vi "FocusLock Control v3.vi"() -> ()   [LabVIEW 2014]
uses:
  Controls/Camera Control.ctl
  Controls/Focus Lock.ctl
  Controls/Standard Action for Camera Control.ctl
  Controls/Standard Action for Focus Lock.ctl
  Controls/Counter Action.ctl
  Controls/Standard Action for Position.ctl
  Controls/StageStates.ctl
  <vilib>/addons/control/pid/pid.llb/PID (DBL Array).vi
  <vilib>/Utility/xml.llb/Write to XML File(string).vi
  <vilib>/Utility/xml.llb/Read From XML File(string).vi
  C:/Program Files (x86)/National Instruments/LabVIEW 2014/instr.lib/IDS/ueye.NET/uEyeDotNet.dll
  Program Files (x86)/National Instruments/LabVIEW 2014/instr.lib/IDS/ueye.NET/uEyeDotNet.dll
  <vilib>/addons/control/pid/NI_PID_pid.lvlib
panel:
  in  "Load":bool
  in  "Save":bool
  out "metric":dbl[](array[numeric])
  in  "Lock Control":T1
  out "Lock Position":cluster{"X":dbl, "Y":dbl, "dx - dy":dbl}
  out "Current Position":cluster{"X":dbl, "Y":dbl, "dx - dy":dbl}
  out "Size difference History":dbl(graph)
  out "Position History":cluster{dbl, dbl}(graph)
  in  "Lock Tolorence":cluster{"XY":dbl, "Z":dbl}={"XY"=0.4, "Z"=0.4}
  out "ROI":u8[][](graph)=[[1, 1, 1, 1, 1, 1, 1, 1, 1, 2, 1, 1, 1, 1, 1, 2, 1, 1, 1, 1, 1, 2, 1, 1, 1, 1, 1, 1, 1, 1, 1, 1, 1, 1, 1, 1, 1, 1, 1, 1, 1, 1, 1, 1, 1, 1, 1, 1, 1, 1], [0, 1, 1, 1, 1, 1, 1, 1, 0, 1, 0, 1, 0, 1, 0, 1, 0, 1, 0, 1, 0, 1, 0, 1, 0, 1, 0, 1, 0, 1, 1, 1, 0, 1, 0, 1, 0, 1, 0, 1, 0, 1, 0, 1, 0, 1, 0, 1, 0, 1], [1, 1, 1, 1, 1, 1, 1, 1, 1, 1, 1, 1, 1, 1, 1, 1, 1, 2, 1, 1, 1, 1, 1, 1, 1, 1, 1, 1, 1, 1, 1, 1, 1, 1, 1, 1, 1, 1, 1, 1, 1, 1, 1, 1, 1, 1, 1, 1, 1, 1], [0, 1, 1, 1, 1, 1, 0, 1, 0, 1, 0, 1, 0, 1, 0, 1, 0, 1, 0, 1, 0, 1, 0, 1, 0, 1, 0, 1, 0, 1, 0, 1, 0, 1, 0, 1, 0, 1, 0, 1, 0, 1, 0, 1, 0, 1, 0, 1, 0, 1], [1, 1, 1, 1, 1, 1, 1, 1, 1, 1, 1, 1, 1, 1, 1, 1, 1, 1, 1, 1, 1, 1, 1, 1, 1, 1, 1, 1, 1, 1, 1, 1, 1, 1, 1, 1, 1, 1, 1, 1, 1, 1, 1, 1, 1, 1, 1, 1, 1, 2], [0, 1, 0, 1, 0, 1, 0, 1, 0, 1, 0, 1, 0, 1, 1, 1, 0, 1, 0, 1, 0, 1, 0, 1, 0, 1, 1, 1, 0, 1, 1, 1, 0, 1, 0, 1, 0, 1, 1, 1, 0, 1, 0, 1, 0, 1, 0, 1, 0, 1], [1, 1, 1, 1, 1, 2, 1, 1, 1, 1, 1, 1, 1, 2, 1, 2, 1, 1, 1, 2, 1, 2, 1, 1, 1, 1, 1, 1, 1, 1, 1, 2, 1, 1, 1, 2, 1, 2, 1, 1, 1, 1, 1, 1, 1, 2, 1, 1, 1, 2], [0, 1, 0, 1, 0, 1, 0, 1, 1, 1, 1, 1, 0, 1, 0, 1, 0, 1, 0, 1, 0, 1, 0, 1, 0, 1, 0, 1, 0, 1, 0, 1, 0, 1, 0, 1, 0, 1, 1, 1, 1, 1, 0, 1, 0, 1, 0, 1, 0, 1], [1, 1, 1, 2, 1, 2, 1, 1, 1, 2, 1, 1, 1, 1, 1, 1, 1, 1, 1, 1, 1, 2, 1, 1, 1, 2, 1, 1, 1, 1, 1, 1, 1, 1, 1, 1, 1, 1, 1, 1, 1, 1, 1, 1, 1, 1, 1, 2, 1, 1], [0, 1, 1, 1, 0, 1, 0, 1, 0, 1, 0, 1, 0, 1, 1, 1, 0, 1, 0, 1, 0, 1, 0, 1, 1, 1, 0, 1, 0, 1, 1, 1, 0, 1, 0, 1, 1, 1, 0, 1, 0, 1, 0, 1, 0, 1, 0, 1, 0, 1], [1, 1, 1, 1, 1, 1, 1, 1, 1, 1, 1, 2, 1, 2, 1, 1, 1, 1, 1, 1, 1, 1, 1, 1, 1, 1, 1, 1, 1, 1, 1, 1, 1, 1, 1, 1, 1, 1, 1, 1, 1, 2, 1, 1, 1, 1, 1, 2, 1, 1], [1, 1, 0, 1, 1, 1, 1, 1, 1, 1, 1, 1, 1, 1, 0, 1, 0, 1, 1, 1, 1, 1, 1, 1, 1, 1, 1, 1, 1, 1, 0, 1, 0, 1, 1, 1, 1, 1, 0, 1, 1, 1, 1, 1, 0, 1, 0, 1, 0, 1], [1, 1, 1, 1, 1, 1, 1, 1, 1, 2, 1, 1, 1, 1, 1, 1, 1, 1, 1, 1, 1, 1, 1, 2, 1, 1, 1, 2, 1, 2, 1, 1, 1, 2, 1, 1, 1, 1, 1, 1, 1, 2, 1, 1, 1, 1, 1, 2, 1, 1], [0, 1, 0, 1, 1, 1, 0, 1, 1, 1, 1, 1, 1, 1, 1, 1, 1, 1, 0, 1, 0, 1, 0, 1, 0, 1, 1, 1, 1, 1, 0, 1, 0, 1, 1, 1, 0, 1, 0, 1, 1, 1, 1, 1, 0, 1, 1, 1, 0, 1], [1, 1, 1, 1, 1, 1, 1, 2, 1, 1, 1, 2, 1, 1, 1, 1, 1, 1, 1, 1, 1, 1, 1, 2, 1, 2, 1, 1, 1, 1, 1, 1, 1, 1, 1, 1, 1, 1, 1, 1, 1, 1, 1, 1, 1, 1, 1, 2, 1, 1], [0, 1, 0, 1, 1, 1, 1, 1, 0, 1, 0, 1, 0, 1, 0, 1, 1, 1, 0, 1, 0, 1, 0, 1, 0, 1, 0, 1, 0, 1, 0, 1, 0, 1, 0, 1, 0, 1, 0, 1, 1, 1, 0, 1, 1, 1, 0, 1, 1, 1], [1, 1, 1, 1, 1, 1, 1, 1, 1, 2, 1, 1, 1, 1, 1, 1, 1, 1, 1, 1, 1, 1, 1, 1, 1, 1, 1, 1, 1, 2, 1, 2, 1, 1, 1, 1, 1, 1, 1, 1, 1, 1, 1, 1, 1, 1, 1, 1, 1, 1], [0, 1, 0, 1, 1, 1, 0, 1, 0, 1, 0, 1, 0, 1, 0, 1, 1, 1, 0, 1, 0, 1, 0, 1, 0, 1, 0, 1, 0, 1, 0, 1, 0, 1, 0, 1, 0, 1, 0, 1, 0, 1, 0, 1, 0, 1, 0, 1, 0, 1], [1, 1, 1, 1, 1, 1, 1, 2, 1, 1, 1, 1, 1, 1, 1, 1, 1, 1, 1, 1, 1, 1, 1, 1, 1, 2, 1, 1, 1, 1, 1, 1, 1, 1, 1, 1, 1, 1, 1, 2, 1, 2, 1, 1, 1, 2, 1, 2, 1, 2], [0, 1, 1, 1, 0, 1, 0, 1, 0, 1, 0, 1, 0, 1, 0, 1, 1, 1, 0, 1, 0, 1, 0, 1, 0, 1, 0, 1, 0, 1, 1, 1, 0, 1, 0, 1, 0, 1, 0, 1, 0, 1, 0, 1, 0, 1, 0, 1, 0, 1], [1, 2, 1, 1, 1, 1, 1, 1, 1, 1, 1, 1, 1, 1, 1, 1, 1, 2, 1, 1, 1, 1, 1, 1, 1, 2, 1, 1, 1, 2, 1, 2, 1, 2, 1, 1, 1, 1, 1, 2, 1, 1, 1, 2, 1, 2, 1, 1, 1, 1], [0, 1, 0, 1, 1, 1, 0, 1, 0, 1, 0, 1, 1, 1, 0, 1, 0, 1, 0, 1, 0, 1, 0, 1, 0, 1, 0, 1, 0, 1, 0, 1, 0, 1, 0, 1, 0, 1, 0, 1, 0, 1, 0, 1, 0, 1, 0, 1, 0, 1], [1, 1, 1, 1, 1, 1, 1, 1, 1, 2, 1, 1, 1, 1, 1, 1, 1, 1, 1, 1, 1, 1, 1, 1, 1, 1, 1, 1, 1, 1, 1, 1, 1, 1, 1, 1, 1, 2, 1, 1, 1, 2, 1, 1, 1, 1, 1, 1, 1, 1], [0, 1, 0, 1, 0, 1, 1, 1, 0, 1, 0, 1, 0, 1, 0, 1, 0, 1, 0, 1, 0, 1, 0, 1, 0, 1, 0, 1, 0, 1, 0, 1, 0, 1, 0, 1, 0, 1, 1, 1, 0, 1, 0, 1, 0, 1, 1, 1, 1, 1], [1, 1, 1, 1, 1, 1, 1, 1, 1, 1, 1, 1, 1, 1, 1, 1, 1, 2, 1, 2, 1, 1, 1, 1, 1, 1, 1, 2, 1, 1, 1, 1, 1, 2, 1, 2, 1, 1, 1, 1, 1, 1, 1, 1, 1, 1, 1, 1, 1, 2], [1, 1, 0, 1, 0, 1, 0, 1, 1, 1, 0, 1, 0, 1, 0, 1, 1, 1, 0, 1, 0, 1, 0, 1, 1, 1, 1, 1, 1, 1, 0, 1, 1, 1, 1, 1, 1, 1, 1, 1, 0, 1, 1, 1, 0, 1, 0, 1, 0, 1], [1, 1, 1, 1, 1, 1, 1, 1, 1, 1, 1, 1, 1, 1, 1, 2, 1, 1, 1, 1, 1, 1, 1, 1, 1, 1, 1, 1, 1, 1, 1, 1, 1, 1, 1, 1, 1, 1, 1, 1, 1, 1, 1, 1, 1, 1, 1, 1, 1, 1], [1, 1, 1, 1, 1, 1, 0, 1, 1, 1, 1, 1, 1, 1, 1, 1, 1, 1, 1, 1, 1, 1, 0, 1, 1, 1, 1, 1, 1, 1, 1, 1, 1, 1, 1, 1, 0, 1, 1, 1, 1, 1, 1, 1, 1, 1, 1, 1, 1, 1], [1, 1, 1, 1, 1, 1, 1, 1, 1, 1, 1, 1, 1, 2, 1, 2, 1, 1, 1, 1, 1, 1, 1, 1, 1, 1, 1, 1, 1, 1, 1, 1, 1, 2, 1, 1, 1, 1, 1, 1, 1, 2, 1, 1, 1, 1, 1, 1, 1, 1], [1, 1, 0, 1, 1, 1, 1, 1, 0, 1, 0, 1, 0, 1, 1, 1, 1, 1, 1, 1, 0, 1, 0, 1, 0, 1, 0, 1, 1, 1, 0, 1, 0, 1, 0, 1, 0, 1, 0, 1, 0, 1, 0, 1, 0, 1, 1, 1, 0, 1], [1, 1, 1, 1, 1, 1, 1, 1, 1, 1, 1, 1, 1, 2, 1, 1, 1, 1, 1, 1, 1, 1, 1, 2, 1, 1, 1, 2, 1, 1, 1, 1, 1, 1, 1, 1, 1, 1, 1, 1, 1, 1, 1, 2, 1, 1, 1, 1, 1, 2], [0, 1, 0, 1, 0, 1, 1, 1, 0, 1, 0, 1, 0, 1, 1, 1, 0, 1, 0, 1, 0, 1, 0, 1, 0, 1, 1, 1, 0, 1, 1, 1, 0, 1, 0, 1, 0, 1, 1, 1, 1, 1, 0, 1, 1, 1, 1, 1, 1, 1], [1, 2, 1, 1, 1, 2, 1, 2, 1, 2, 1, 1, 1, 2, 1, 1, 1, 1, 1, 1, 1, 1, 1, 1, 1, 1, 1, 1, 1, 2, 1, 1, 1, 1, 1, 1, 1, 2, 1, 1, 1, 1, 1, 1, 1, 1, 1, 1, 1, 1], [0, 1, 0, 1, 0, 1, 0, 1, 1, 1, 1, 1, 1, 1, 1, 1, 1, 1, 0, 1, 0, 1, 0, 1, 0, 1, 0, 1, 0, 1, 0, 1, 0, 1, 0, 1, 0, 1, 0, 1, 0, 1, 1, 1, 0, 1, 0, 1, 0, 1], [1, 1, 1, 1, 1, 1, 1, 1, 1, 1, 1, 1, 1, 1, 1, 1, 1, 1, 1, 2, 1, 2, 1, 1, 1, 1, 1, 1, 1, 1, 1, 1, 1, 1, 1, 1, 1, 1, 1, 1, 1, 1, 1, 1, 1, 1, 1, 1, 1, 1], [0, 1, 1, 1, 1, 1, 0, 1, 0, 1, 0, 1, 1, 1, 0, 1, 0, 1, 0, 1, 1, 1, 0, 1, 0, 1, 0, 1, 0, 1, 0, 1, 0, 1, 0, 1, 0, 1, 1, 1, 0, 1, 0, 1, 0, 1, 0, 1, 1, 1], [1, 1, 1, 1, 1, 1, 1, 1, 1, 1, 1, 1, 1, 1, 1, 1, 1, 1, 1, 1, 1, 1, 1, 1, 1, 2, 1, 1, 1, 2, 1, 1, 1, 1, 1, 2, 1, 2, 1, 2, 1, 1, 1, 1, 1, 1, 1, 1, 1, 1], [0, 1, 1, 1, 1, 1, 0, 1, 0, 1, 0, 1, 1, 1, 0, 1, 0, 1, 0, 1, 0, 1, 0, 1, 0, 1, 0, 1, 1, 1, 1, 1, 0, 1, 0, 1, 0, 1, 1, 1, 0, 1, 1, 1, 0, 1, 0, 1, 0, 1], [1, 1, 1, 1, 1, 1, 1, 1, 1, 1, 1, 1, 1, 1, 1, 1, 1, 1, 1, 1, 1, 1, 1, 2, 1, 1, 1, 2, 1, 1, 1, 2, 1, 1, 1, 2, 1, 1, 1, 2, 1, 1, 1, 1, 1, 1, 1, 1, 1, 1], [0, 1, 0, 1, 0, 1, 0, 1, 0, 1, 1, 1, 0, 1, 0, 1, 0, 1, 1, 1, 0, 1, 0, 1, 0, 1, 1, 1, 1, 1, 1, 1, 0, 1, 0, 1, 1, 1, 0, 1, 0, 1, 0, 1, 1, 1, 1, 1, 1, 1], [1, 1, 1, 1, 1, 1, 1, 1, 1, 1, 2, 1, 1, 1, 1, 1, 1, 1, 1, 1, 2, 1, 1, 1, 1, 1, 1, 1, 1, 1, 1, 1, 1, 1, 1, 1, 1, 1, 1, 1, 1, 1, 1, 1, 1, 1, 1, 1, 1, 1], [1, 1, 0, 1, 0, 1, 0, 1, 0, 1, 0, 1, 1, 1, 0, 1, 0, 1, 0, 1, 0, 1, 1, 1, 0, 1, 0, 1, 0, 1, 0, 1, 0, 1, 0, 1, 0, 1, 0, 1, 0, 1, 0, 1, 0, 1, 0, 1, 0, 1], [1, 1, 1, 1, 1, 1, 1, 1, 1, 1, 1, 1, 1, 1, 1, 1, 1, 1, 1, 1, 1, 1, 1, 1, 1, 1, 1, 1, 1, 1, 1, 1, 1, 1, 1, 1, 1, 1, 1, 1, 1, 1, 1, 1, 1, 1, 1, 2, 1, 1], [0, 1, 1, 1, 0, 1, 0, 1, 0, 1, 0, 1, 0, 1, 0, 1, 0, 1, 0, 1, 0, 1, 0, 1, 0, 1, 0, 1, 0, 1, 0, 1, 0, 1, 0, 1, 0, 1, 0, 1, 0, 1, 0, 1, 0, 1, 0, 1, 0, 1], [1, 1, 1, 1, 1, 1, 1, 1, 1, 1, 1, 1, 1, 1, 1, 1, 1, 1, 1, 1, 1, 1, 1, 1, 1, 1, 1, 1, 1, 1, 1, 1, 1, 1, 1, 1, 1, 1, 1, 1, 1, 1, 1, 1, 1, 1, 1, 1, 1, 2], [0, 1, 0, 1, 0, 1, 0, 1, 0, 1, 0, 1, 0, 1, 0, 1, 0, 1, 1, 1, 0, 1, 0, 1, 0, 1, 0, 1, 0, 1, 0, 1, 0, 1, 0, 1, 0, 1, 0, 1, 0, 1, 0, 1, 0, 1, 0, 1, 0, 1], [1, 1, 1, 1, 1, 1, 1, 1, 1, 1, 1, 1, 1, 1, 1, 1, 1, 1, 1, 1, 1, 1, 1, 1, 1, 1, 1, 2, 1, 2, 1, 2, 1, 1, 1, 1, 1, 1, 1, 2, 1, 1, 1, 1, 1, 1, 1, 1, 1, 1], [0, 1, 0, 1, 0, 1, 0, 1, 0, 1, 0, 1, 0, 1, 0, 1, 0, 1, 0, 1, 0, 1, 0, 1, 0, 1, 0, 1, 0, 1, 0, 1, 0, 1, 0, 1, 0, 1, 0, 1, 0, 1, 0, 1, 0, 1, 0, 1, 0, 1], [1, 1, 1, 1, 1, 1, 1, 1, 1, 1, 1, 1, 1, 1, 1, 2, 1, 1, 1, 1, 1, 1, 1, 1, 1, 1, 1, 1, 1, 2, 1, 1, 1, 2, 1, 1, 1, 1, 1, 2, 1, 1, 1, 1, 1, 1, 1, 2, 1, 1], [0, 1, 0, 1, 0, 1, 0, 1, 0, 1, 1, 1, 0, 1, 0, 1, 0, 1, 0, 1, 0, 1, 0, 1, 0, 1, 0, 1, 1, 1, 0, 1, 0, 1, 0, 1, 0, 1, 1, 1, 0, 1, 1, 1, 0, 1, 0, 1, 1, 1]]
  in  "Camera Control":T2={"Pixel Clock (MHz)"=0, "Exposure Time (ms)"=0.0, "Frame Rate (fps)"=10.000850072256142, "ROI Half Width"=100, "Switch"=TRUE} {"Frame Rate (fps)" scale=6.1..17.45; "Exposure Time (ms)" scale=0.06..1.0; "Pixel Clock (MHz)" scale=5.0..43.0}
  out "Camera Image":u8[][](graph)
  in  "Laser Control":refnum<k7>(container)
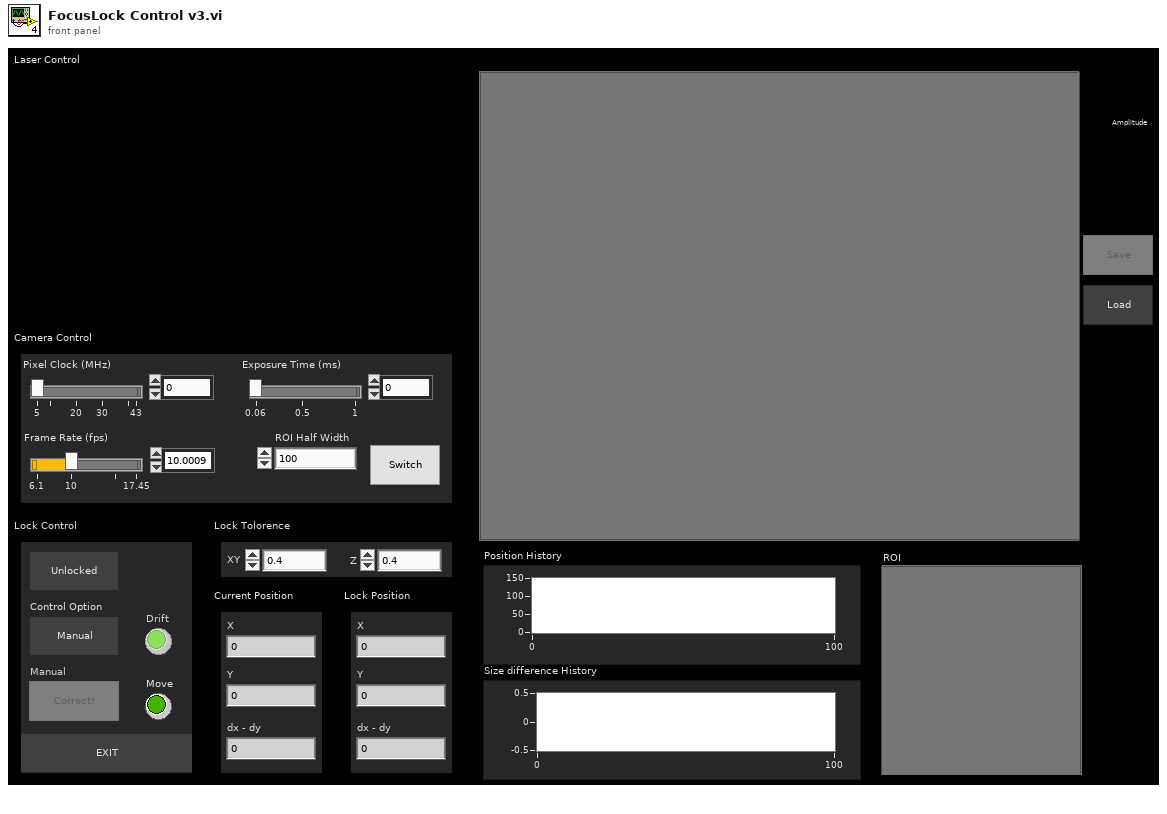
[diagram p1: front panel]
types:
  T1 = typedef "Focus Lock.ctl" = cluster{"EXIT":bool, "Lock Current":bool, "Manual":bool, "Drift":bool, "Move":bool, "Control Option":bool}
  T2 = typedef "Camera Control.ctl" = cluster{"Pixel Clock (MHz)":i32, "Exposure Time (ms)":dbl, "Frame Rate (fps)":dbl, "ROI Half Width":i32, "Switch":bool}
  T3 = typedef "Standard Action for Camera Control.ctl" = enum16{"Read", "Setting", "Switch", "Initialization", "Exit"}
  T4 = typedef "Standard Action for Focus Lock.ctl" = enum16{"Read", "Write"}
  T5 = typedef "Counter Action.ctl" = enum16{"Zero", "Plus One", "Read"}
  T6 = enum8{"Enabled", "Disabled", "Disabled and Grayed Out"}
  T7 = typedef "Standard Action for Position.ctl" = enum16{"Read", "Write Current", "Write Lock"}
  T8 = typedef "LVPointDoubleTypeDef.ctl" = cluster{"Cursor X":dbl, "Cursor Y":dbl}
  T9 = cluster{"Cursor.Cursor X":dbl, "Cursor.Cursor Y":dbl, "Lock Position":cluster{"X":dbl, "Y":dbl, "dx - dy":dbl}, "Lock Control  out":T1}
  T10 = cluster{"proportional gain (Kc)":dbl, "integral time (Ti, min)":dbl, "derivative time (Td, min)":dbl}[]
  T11 = typedef "StageStates.ctl" = enum16{"POSITION", "MVR", "MOVE", "HALT", "ONTARGET", "ERROR", "EXIT", "HOME", "ZEROPOS", "NANOPOS", "QUIT", "ANALOG"}
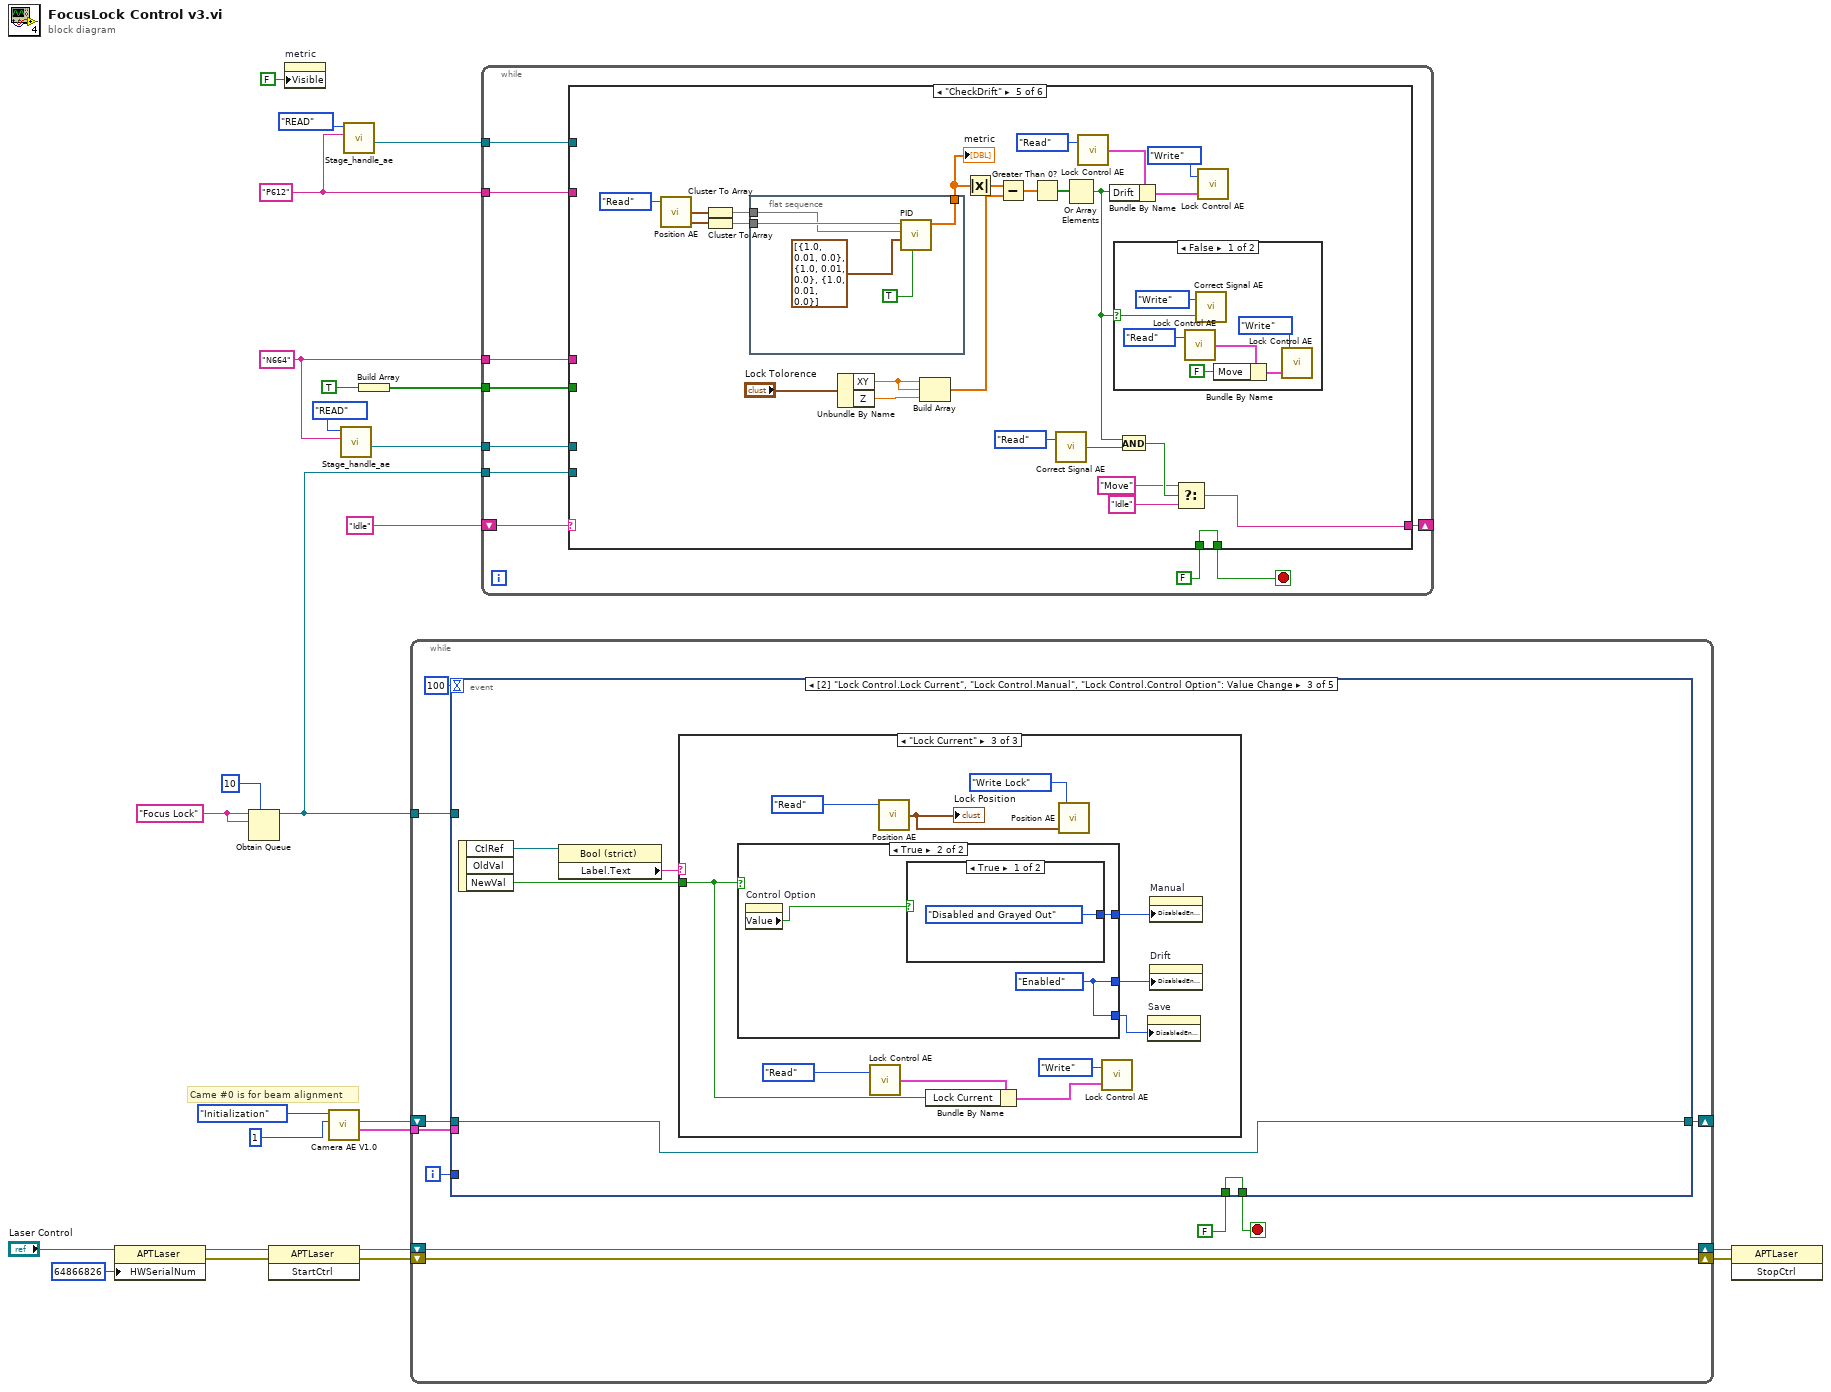
[diagram p0: block diagram]
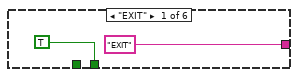
[diagram p2: hidden frame]
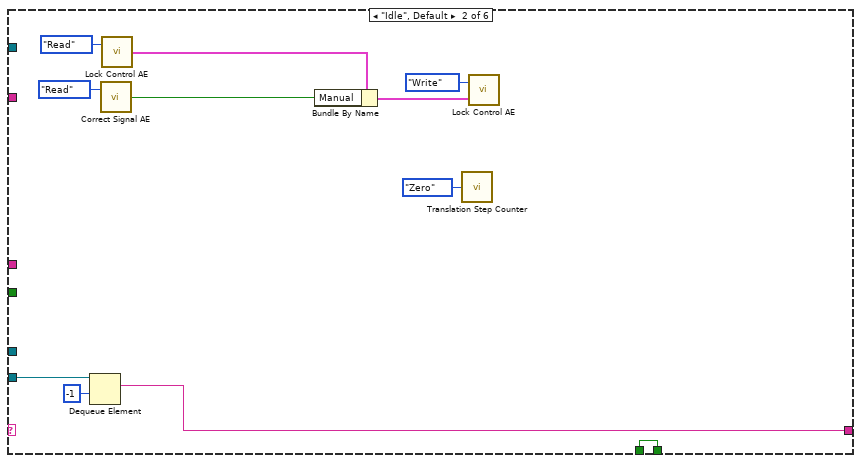
[diagram p3: hidden frame]
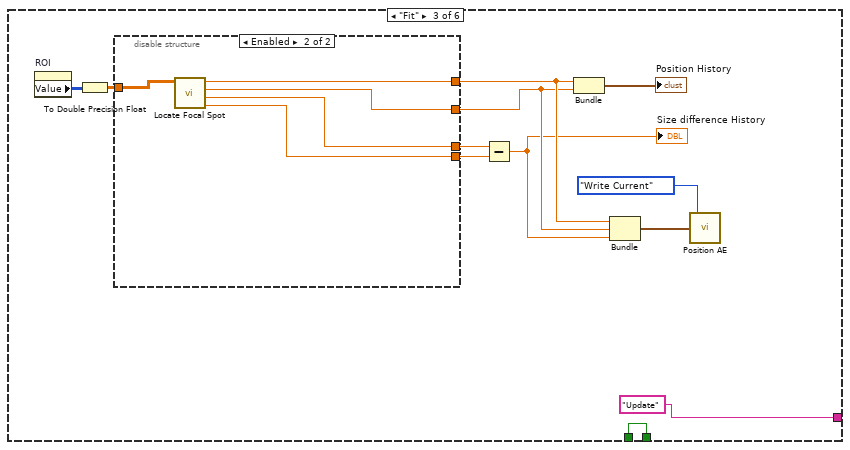
[diagram p4: hidden frame]
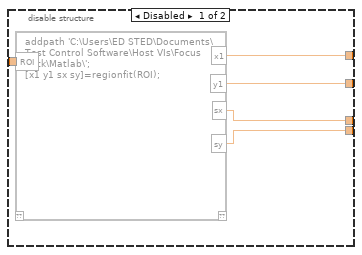
[diagram p5: hidden frame]
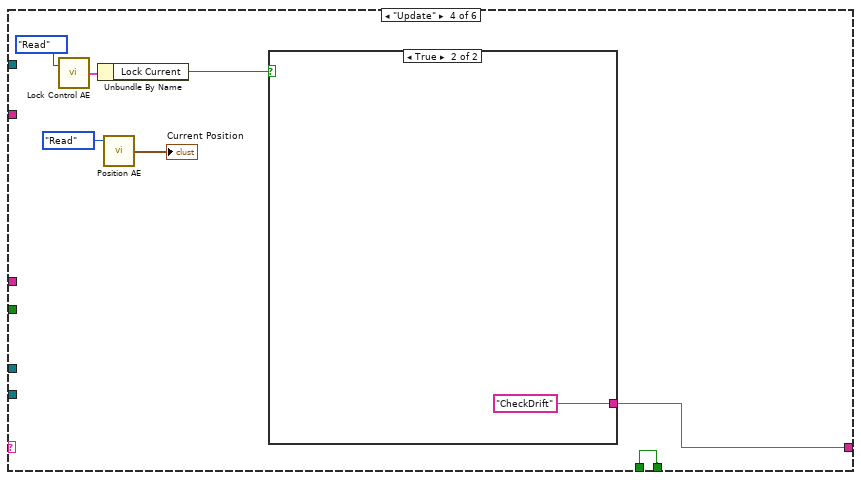
[diagram p6: hidden frame]
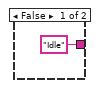
[diagram p7: hidden frame]
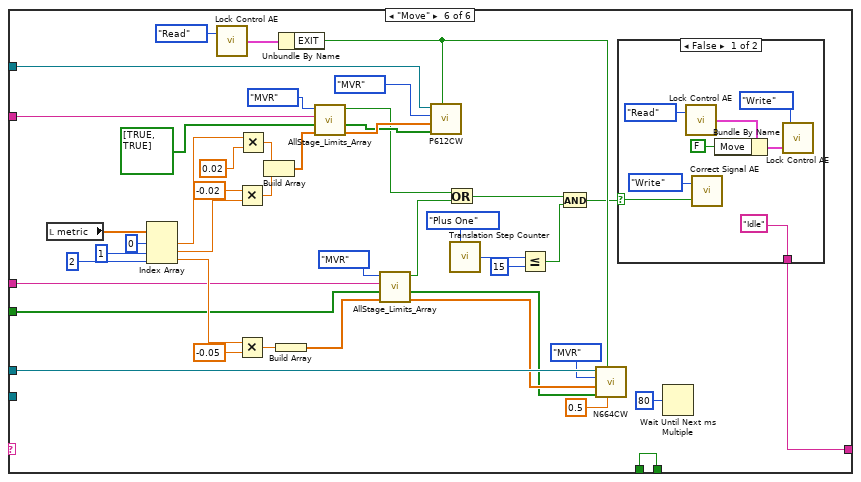
[diagram p9: hidden frame]
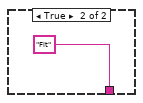
[diagram p10: hidden frame]
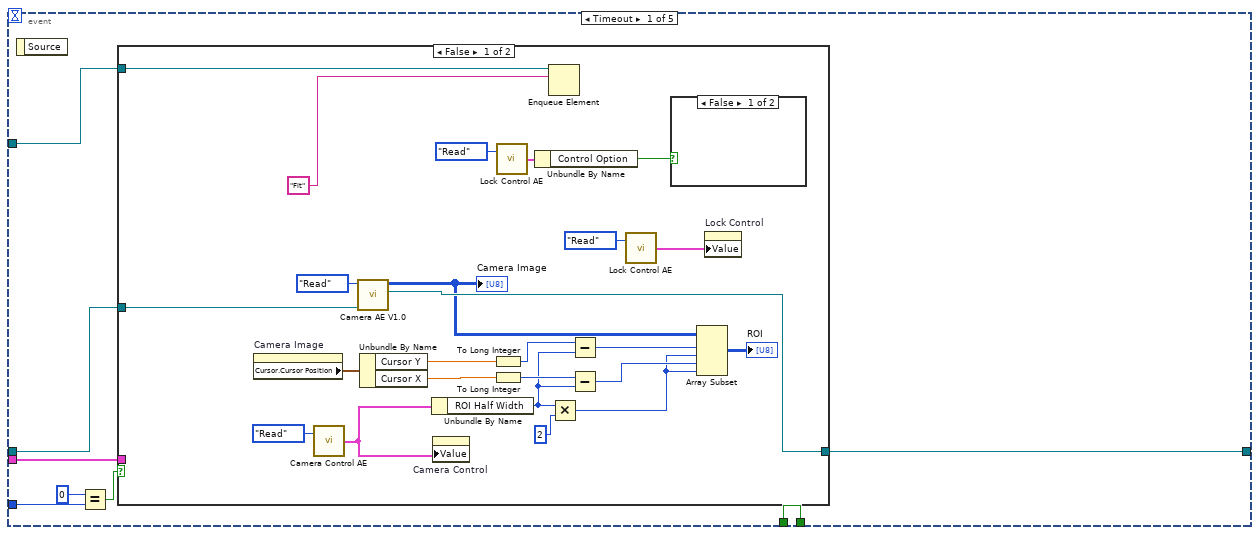
[diagram p11: hidden frame]
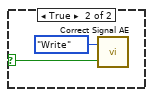
[diagram p12: hidden frame]
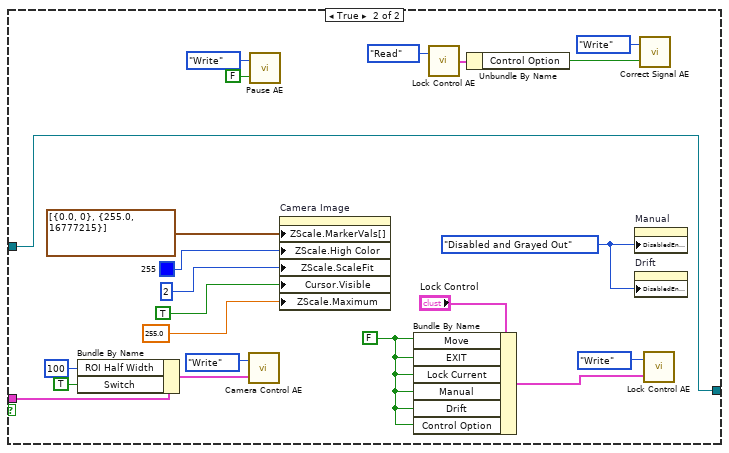
[diagram p13: hidden frame]
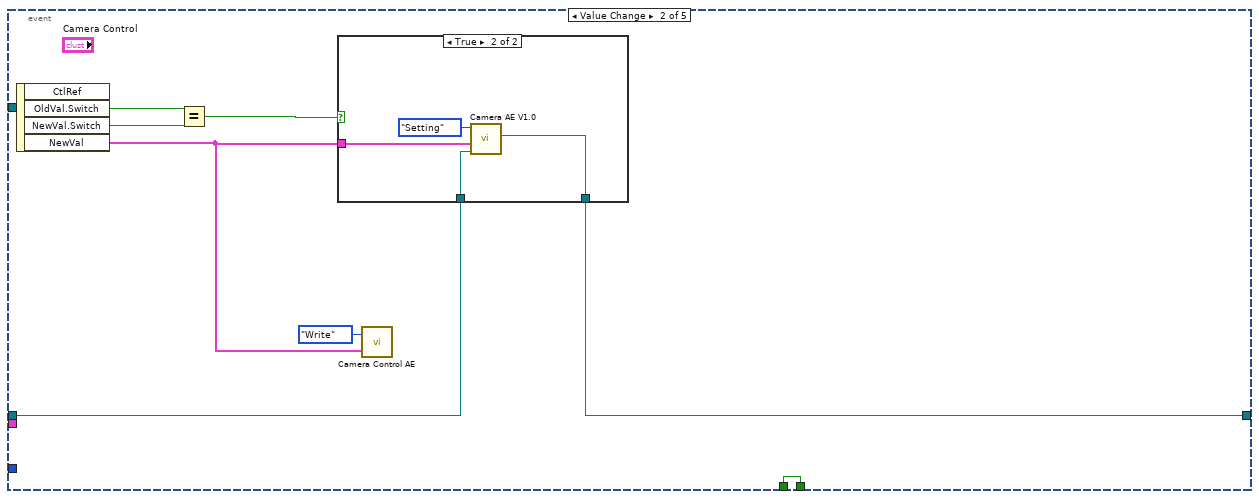
[diagram p14: hidden frame]
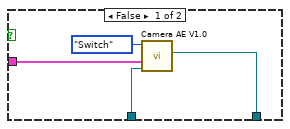
[diagram p15: hidden frame]
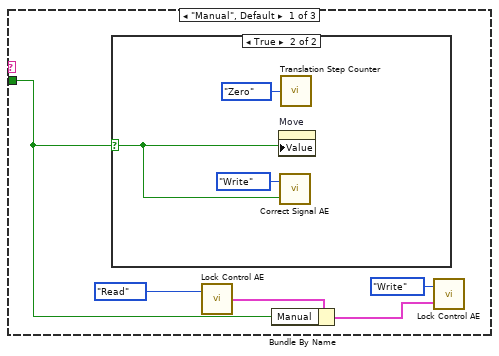
[diagram p16: hidden frame]
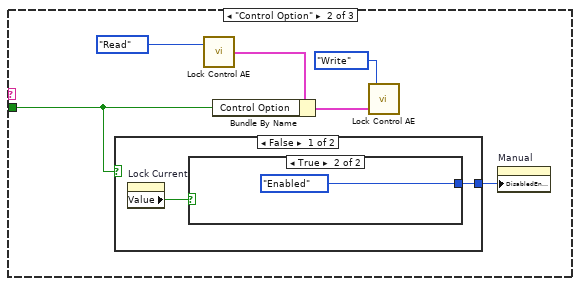
[diagram p18: hidden frame]
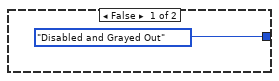
[diagram p19: hidden frame]
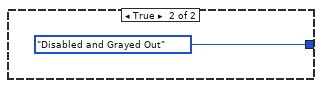
[diagram p20: hidden frame]
diagram:
  w9 = "N664" ("StageID")
  w12 = "P612" ("StageID")
  w16 = "Focus Lock" ("name (unnamed)")
  # "Came #0 is for beam alignment"
  n1 = property class="APTLaser"(reference="Laser Control", "HWSerialNum"=64866826) -> (reference out=w23:refnum<k7>, error out=w22:errorcluster)  [unwired: 1 in]
  n2 = Obtain Queue(max queue size (-1, unlimited)=10, name (unnamed)=w16, element data type=w16) -> (queue out=w14:refnum<queue>)  [unwired: 2 in, 2 out]
  n3 = invoke class="APTLaser" method="StartCtrl"(reference=w23, error in=w22) -> (reference out=w21:refnum<k7>, error out=w19:errorcluster)  [unwired: 1 in, 1 out]
  n4 = property on="metric" class="Arr (strict)"("Visible"=FALSE) -> ()  [unwired: 2 in, 2 out]
  n5 = call "Camera AE V1.0.vi"("Camera ID"=1, "Action"=Standard_Action_for_Camera_Control."Initialization") -> ("Camera Control Out"=w17:T2, "Reference Out"=w1:refnum<k24>)  [unwired: 4 in, 2 out]
  n6 = call "Stage_handle_ae.vi"("StageID"=w9, "Enum"=enum16{"WRITE", "READ"}."READ") -> ("Visa Out"=w7:refnum<visa-resource-name>)  [unwired: 9 in]
  n7 = call "Stage_handle_ae.vi"("StageID"=w12, "Enum"=enum16{"WRITE", "READ"}."READ") -> ("Visa Out"=w10:refnum<visa-resource-name>)  [unwired: 9 in]
  n8 = Build Array(TRUE) -> (w4:bool[])
  n9 = while {
    shift-right: [w35] -> w20
    shift-left: w21 -> [w35]
    shift-right: [w34] -> w18
    shift-left: w19 -> [w34]
    tunnel: w17 -> [w29]
    tunnel: w14 -> [w28]
    shift-right: [w26] -> _
    shift-left: w1 -> [w27]
    i -> [w31]
    stop <- w32 stop-if-true
    n10 = event shown="[2] \"Lock Control.Lock Current\", \"Lock Control.Manual\", \"Lock Control.Control Option\": Value Change" {
      selector: _ -> [_ _ _ _ _]
      dyn-events: _ -> [_ _ _ _ _]
      timeout: 100 -> [_ _ _ _ _]
      tunnel: FALSE -> [w43 w99 w109 w156 _]
      tunnel: [w43 w99 w109 w156 w206] -> w32
      tunnel: w31 -> [w42 _ _ _ _]
      tunnel: w29 -> [w39 _ _ _ _]
      tunnel: w28 -> [w37 _ _ w152 w209]
      tunnel: w27 -> [w38 w93 w108 w154 w205]
      tunnel: [w36 w92 w108 w154 _] -> w26
      event Timeout {
        n11 = event-data() -> ()  [unwired: 1 in, 1 out]
        n12 = Equal?(x=0, y=w42) -> (x = y?=w40:bool)
        n13 = case shown="False" w40 {
          tunnel: w39 -> [_ w85]
          tunnel: w38 -> [w67 w76]
          tunnel: w37 -> [w66 _]
          tunnel: [w64 w76] -> w36
          frame False {
            n14 = property on="Camera Image" class="IntGraph (strict)"() -> ("Cursor.Cursor Position"=w60:T8)  [unwired: 2 in, 2 out]
            n15 = call "Camera Control AE.vi"("Action"=Standard_Action_for_Focus_Lock."Read") -> ("Camera Control Output"=w47:T2)  [unwired: 1 in]
            n16 = call "Camera AE V1.0.vi"(".NET (Reference)"=w67, "Action"=Standard_Action_for_Camera_Control."Read") -> ("Reference Out"=w64:refnum<k24>, "Array"=w58:u8[][])  [unwired: 4 in, 2 out]
            "Camera Image" <- w58
            n17 = Unbundle By Name(w60) -> ("Cursor Y"=w57:dbl, "Cursor X"=w56:dbl)
            n18 = Unbundle By Name(w47) -> ("ROI Half Width"=w52:i32)
            n19 = property on="Camera Control" class="Clust (strict)"("Value"=w47) -> ()  [unwired: 2 in, 2 out]
            n20 = To Long Integer(number=w57) -> (32bit integer=w54:i32)
            n21 = To Long Integer(number=w56) -> (32bit integer=w53:i32)
            n22 = call "Lock Control AE.vi"("Action"=Standard_Action_for_Focus_Lock."Read") -> ("Lock Control  out"=w45:T1)  [unwired: 1 in]
            n23 = Unbundle By Name(w45) -> ("Control Option"=w44:bool)
            n24 = Enqueue Element(queue=w66, element="Fit") -> ()  [unwired: 2 in, 3 out]
            n25 = Multiply(x=w52, y=2) -> (x*y=w49:i32)
            n26 = Subtract(x=w54, y=w52) -> (x-y=w51:i32)
            n27 = Subtract(x=w53, y=w52) -> (x-y=w50:i32)
            n28 = call "Lock Control AE.vi"("Action"=Standard_Action_for_Focus_Lock."Read") -> ("Lock Control  out"=w62:T1)  [unwired: 1 in]
            n29 = case shown="False" w44 {
              selector: w44 -> [_ w68]
              frame False {
              }
              frame True {
                n30 = call "Correct Signal AE.vi"("signal in"=w68, "Action"=Standard_Action_for_Focus_Lock."Write") -> ()  [unwired: 1 out]
              }
            }
            n31 = Array Subset(array=w58, index (row)=w51, length (row)=w49, index (col)=w50, length (col)=w49) -> (→"ROI":u8[][])
            n32 = property on="Lock Control" class="Clust"("Value"=w62) -> ()  [unwired: 2 in, 2 out]
          }
          frame True {
            w78 = T6."Disabled and Grayed Out" ("Disabled")
            w70 = FALSE ("EXIT")
            n33 = Bundle By Name(cluster=w85, "ROI Half Width"=100, "Switch"=TRUE) -> (w83:T2)
            n34 = call "Camera Control AE.vi"("Camera Control Input"=w83, "Action"=Standard_Action_for_Focus_Lock."Write") -> ()  [unwired: 1 out]
            n35 = call "Pause AE.vi"("Pause In"=FALSE, "Action"=Standard_Action_for_Focus_Lock."Write") -> ()  [unwired: 1 out]
            n36 = property on="Camera Image" class="IntGraph (strict)"("ZScale.MarkerVals[]"=cluster{dbl, u32}[] [{0.0, 0}, {255.0, 16777215}] ("Z Scale.Marker Values[]"), "ZScale.High Color"=u32 255, "ZScale.ScaleFit"=u8 2 ("Z Scale.Scale Fit"), "Cursor.Visible"=TRUE, "ZScale.Maximum"=255.0 ("Z Scale.Range:Maximum")) -> ()  [unwired: 2 in, 2 out]
            n37 = Bundle By Name(cluster="Lock Control", "Move"=w70, "EXIT"=w70, "Lock Current"=w70, "Manual"=w70, "Drift"=w70, "Control Option"=w70) -> (w79:T1)
            n38 = call "Lock Control AE.vi"("Action"=Standard_Action_for_Focus_Lock."Read") -> ("Lock Control  out"=w72:T1)  [unwired: 1 in]
            n39 = Unbundle By Name(w72) -> ("Control Option"=w71:bool)
            n40 = property on="Manual" class="Bool (strict)"("DisabledEnum"=w78) -> ()  [unwired: 2 in, 2 out]
            n41 = property on="Drift" class="Bool (strict)"("DisabledEnum"=w78) -> ()  [unwired: 2 in, 2 out]
            n42 = call "Correct Signal AE.vi"("signal in"=w71, "Action"=Standard_Action_for_Focus_Lock."Write") -> ()  [unwired: 1 out]
            n43 = call "Lock Control AE.vi"("Lock Control  in"=w79, "Action"=Standard_Action_for_Focus_Lock."Write") -> ()  [unwired: 1 out]
          }
        }
      }
      event Value Change {
        n44 = event-data() -> ("OldVal.Switch"=w97:bool, "NewVal.Switch"=w96:bool, "NewVal"=w95:T2)  [unwired: 1 in, 1 out]
        n45 = Equal?(x=w97, y=w96) -> (x = y?=w94:bool)
        n46 = case shown="True" w94 {
          tunnel: w95 -> [w103 w106]
          tunnel: w93 -> [w101 w104]
          tunnel: [w100 w105] -> w92
          frame False {
            n47 = call "Camera AE V1.0.vi"(".NET (Reference)"=w101, "Camera Control In"=w103, "Action"=Standard_Action_for_Camera_Control."Switch") -> ("Reference Out"=w100:refnum<k24>)  [unwired: 3 in, 3 out]
          }
          frame True {
            n48 = call "Camera AE V1.0.vi"(".NET (Reference)"=w104, "Camera Control In"=w106, "Action"=Standard_Action_for_Camera_Control."Setting") -> ("Reference Out"=w105:refnum<k24>)  [unwired: 3 in, 3 out]
          }
        }
        n49 = call "Camera Control AE.vi"("Camera Control Input"=w95, "Action"=Standard_Action_for_Focus_Lock."Write") -> ()  [unwired: 1 out]
      }
      event Value Change {
        n50 = event-data() -> ("CtlRef"=w112:refnum<vi>, "NewVal"=w110:bool)  [unwired: 1 in, 1 out]
        n51 = property class="Bool (strict)"(reference=w112) -> ("Label.Text"=w111:string)  [unwired: 1 in, 2 out]
        n52 = case shown="\"Lock Current\"" w111 {
          tunnel: w110 -> [w113 w122 w134]
          frame "Manual", Default {
            n53 = case shown="True" w113 {
              selector: w113 -> [_ w119]
              frame False {
              }
              frame True {
                n54 = property on="Move" class="Bool (strict)"("Value"=w119) -> ()  [unwired: 2 in, 2 out]
                n55 = call "Correct Signal AE.vi"("signal in"=w119, "Action"=Standard_Action_for_Focus_Lock."Write") -> ()  [unwired: 1 out]
                n56 = call "Translation Step Counter.vi"("Action"=Counter_Action."Zero") -> ()  [unwired: 1 out]
              }
            }
            n57 = call "Lock Control AE.vi"("Action"=Standard_Action_for_Focus_Lock."Read") -> ("Lock Control  out"=w116:T1)  [unwired: 1 in]
            n58 = Bundle By Name(cluster=w116, "Manual"=w113) -> (w115:T1)
            n59 = call "Lock Control AE.vi"("Lock Control  in"=w115, "Action"=Standard_Action_for_Focus_Lock."Write") -> ()  [unwired: 1 out]
          }
          frame "Control Option" {
            n60 = case shown="False" w122 {
              tunnel: [w128 T6."Disabled and Grayed Out" ("Disabled")] -> w121
              frame False {
                n61 = property on="Lock Current" class="Bool (strict)"() -> ("Value"=w127:bool)  [unwired: 2 in, 2 out]
                n62 = case shown="True" w127 {
                  tunnel: [T6."Disabled and Grayed Out" ("Disabled") T6."Enabled" ("Disabled")] -> w128
                  frame False {
                  }
                  frame True {
                  }
                }
              }
              frame True {
              }
            }
            n63 = call "Lock Control AE.vi"("Action"=Standard_Action_for_Focus_Lock."Read") -> ("Lock Control  out"=w125:T1)  [unwired: 1 in]
            n64 = Bundle By Name(cluster=w125, "Control Option"=w122) -> (w124:T1)
            n65 = call "Lock Control AE.vi"("Lock Control  in"=w124, "Action"=Standard_Action_for_Focus_Lock."Write") -> ()  [unwired: 1 out]
            n66 = property on="Manual" class="Bool (strict)"("DisabledEnum"=w121) -> ()  [unwired: 2 in, 2 out]
          }
          frame "Lock Current" {
            n67 = case shown="True" w134 {
              tunnel: [w143 w146] -> w142
              tunnel: [w143 w144] -> w133
              tunnel: [w143 w144] -> w132
              frame False {
                w143 = T6."Disabled and Grayed Out" ("Disabled")
              }
              frame True {
                w144 = T6."Enabled" ("Disabled")
                n68 = property on="Control Option" class="Bool (strict)"() -> ("Value"=w145:bool)  [unwired: 2 in, 2 out]
                n69 = case shown="True" w145 {
                  tunnel: [T6."Disabled and Grayed Out" ("Disabled") T6."Enabled" ("Disabled")] -> w146
                  frame True {
                  }
                  frame False {
                  }
                }
              }
            }
            n70 = call "Lock Control AE.vi"("Action"=Standard_Action_for_Focus_Lock."Read") -> ("Lock Control  out"=w137:T1)  [unwired: 1 in]
            n71 = call "Position AE.vi"("Action"=Standard_Action_for_Position."Read") -> ("Current Position out"=w140:cluster{"X":dbl, "Y":dbl, "dx - dy":dbl})  [unwired: 3 in, 1 out]
            "Lock Position" <- w140
            n72 = Bundle By Name(cluster=w137, "Lock Current"=w134) -> (w136:T1)
            n73 = call "Position AE.vi"("Locked Position in"=w140, "Action"=Standard_Action_for_Position."Write Lock") -> ()  [unwired: 2 in, 2 out]
            n74 = call "Lock Control AE.vi"("Lock Control  in"=w136, "Action"=Standard_Action_for_Focus_Lock."Write") -> ()  [unwired: 1 out]
            n75 = property on="Save" class="Bool"("DisabledEnum"=w132) -> ()  [unwired: 2 in, 2 out]
            n76 = property on="Manual" class="Bool (strict)"("DisabledEnum"=w142) -> ()  [unwired: 2 in, 2 out]
            n77 = property on="Drift" class="Bool (strict)"("DisabledEnum"=w133) -> ()  [unwired: 2 in, 2 out]
          }
        }
      }
      event "Save", "Load": Value Change {
        n78 = event-data() -> ("CtlRef"=w157:refnum<vi>)  [unwired: 1 in]
        n79 = control-ref of="Lock Control"() -> (w153:refnum<vi>)
        n80 = call "Lock Control AE.vi"() -> ("Lock Control  out"=w151:T1)  [unwired: 2 in]
        n81 = property class="Bool"(reference=w157) -> ("Label.Text"=w155:string)  [unwired: 1 in, 2 out]
        n82 = property class="Clust"(reference=w153) -> ("Value"=w150:variant)  [unwired: 1 in, 2 out]
        n83 = Variant To Data(type=w151, Variant=w150) -> (data=w149:T1)  [unwired: 1 in, 1 out]
        n84 = case shown="\"Load\"" w155 {
          tunnel: w152 -> [_ _ w172]
          tunnel: w149 -> [_ w158 w171]
          frame Default {
          }
          frame "Save" {
            n85 = control-ref of="Camera Image"() -> (w164:refnum<vi>)
            n86 = property class="IntGraph (strict)"(reference=w164) -> ("Cursor.Cursor X"=w161:dbl, "Cursor.Cursor Y"=w160:dbl)  [unwired: 1 in, 2 out]
            n87 = local read "Lock Position"() -> (w163:cluster{"X":dbl, "Y":dbl, "dx - dy":dbl})
            n88 = call "File Dialog"("start path"=path "C:/Users/ED STED/Documents/Test Control Software/Host VIs/Focus Lock/Data") -> ("selected path"=w162:path, "error out"=w165:errorcluster)  [unwired: 11 in, 2 out]
            n89 = Bundle("Cursor.Cursor X"=w161, "Cursor.Cursor Y"=w160, "Lock Position"=w163, "Lock Control  out"=w158) -> (w159:T9)  [unwired: 1 in]
            n90 = case shown="No Error" w165 {
              tunnel: w162 -> [w169 _]
              tunnel: w159 -> [w168 _]
              frame No Error {
                n91 = Flatten To XML(anything=w168) -> (xml string=w167:string)
                n92 = call-poly <vilib>:"Write to XML File.vi"("XML Input"=w167, "XML File Path"=w169) -> ()  [unwired: 7 in, 3 out]
              }
              frame Error {
                n93 = One Button Dialog(message="\"Incorrect File Input, or no  \nfile is selected! Try again!\"") -> ()  [unwired: 1 in, 1 out]
              }
            }
          }
          frame "Load" {
            n94 = control-ref of="Camera Image"() -> (w174:refnum<vi>)
            n95 = call "File Dialog2"("start path"=path "C:/Users/ED STED/Documents/Test Control Software/Host VIs/Focus Lock/Data") -> ("selected path"=w181:path, "error out"=w180:errorcluster)  [unwired: 11 in, 2 out]
            n96 = property class="IntGraph (strict)"(reference=w174) -> ("Cursor.Cursor X"=w176:dbl, "Cursor.Cursor Y"=w175:dbl)  [unwired: 1 in, 2 out]
            n97 = local read "Lock Position"() -> (w173:cluster{"X":dbl, "Y":dbl, "dx - dy":dbl})
            n98 = call-poly <vilib>:"Read From XML File.vi"("error in (no error)"=w180, "XML File Path"=w181) -> ("error out"=w179:errorcluster, "XML Elements"=w177:string)  [unwired: 7 in, 1 out]
            n99 = Bundle("Cursor.Cursor X"=w176, "Cursor.Cursor Y"=w175, "Lock Position"=w173, "Lock Control  out"=w171) -> (w178:T9)  [unwired: 1 in]
            n100 = case shown="No Error" w179 {
              tunnel: w178 -> [w191 _]
              tunnel: w177 -> [w193 _]
              tunnel: w174 -> [w190 _]
              tunnel: w172 -> [w184 _]
              frame No Error {
                n101 = Unflatten From XML(xml string=w193, type=w191) -> (value=w192:T9)  [unwired: 1 in, 1 out]
                n102 = Unbundle By Name(w192) -> ("Lock Position"=w188:cluster{"X":dbl, "Y":dbl, "dx - dy":dbl}, "Lock Control  out"=w183:T1, "Cursor.Cursor X"=w186:dbl, "Cursor.Cursor Y"=w187:dbl)
                n103 = local write "Lock Position"(w188) -> ()
                n104 = property class="IntGraph (strict)"(reference=w190, "Cursor.Cursor X"=w186, "Cursor.Cursor Y"=w187) -> ()  [unwired: 1 in, 2 out]
                n105 = call "Position AE.vi"("Locked Position in"=w188, "Action"=Standard_Action_for_Position."Write Lock") -> ()  [unwired: 2 in, 2 out]
                n106 = flat-sequence {
                  tunnel: w183 -> [w198]
                  tunnel: [w194] -> w185
                  tunnel: w184 -> [w194]
                  tunnel: w185 -> [w203]
                  frame #0 {
                    w195 = T6."Enabled" ("Disabled")
                    n107 = call "Lock Control AE.vi"("Lock Control  in"=w198, "Action"=Standard_Action_for_Focus_Lock."Write") -> ()  [unwired: 1 out]
                    n108 = control-ref of="Manual"() -> (w197:refnum<vi>)
                    n109 = control-ref of="Drift"() -> (w196:refnum<vi>)
                    n110 = property class="Bool (strict)"(reference=w197, "DisabledEnum"=w195) -> ()  [unwired: 1 in, 2 out]
                    n111 = property class="Bool (strict)"(reference=w196, "DisabledEnum"=w195) -> ()  [unwired: 1 in, 2 out]
                  }
                  frame #1 {
                    n112 = call "Correct Signal AE.vi"("signal in"=TRUE, "Action"=Standard_Action_for_Focus_Lock."Write") -> ()  [unwired: 1 out]
                    n113 = Enqueue Element(queue=w203, element="Fit") -> ()  [unwired: 2 in, 3 out]
                  }
                }
              }
              frame Error {
                n114 = One Button Dialog(message="\"Incorrect File Input, or no  \nfile is selected! Try again!\"") -> ()  [unwired: 1 in, 1 out]
              }
            }
          }
        }
      }
      event Value Change {
        n115 = event-data() -> ("NewVal"=w206:bool)  [unwired: 1 in]
        n116 = call "Camera AE V1.0.vi"(".NET (Reference)"=w205, "Action"=Standard_Action_for_Camera_Control."Exit") -> ()  [unwired: 4 in, 4 out]
        n117 = Enqueue Element(queue=w209, element="EXIT") -> ()  [unwired: 2 in, 3 out]
      }
    }
  }
  n118 = while {
    tunnel: w14 -> [w219]
    shift-right: [w218] -> _
    shift-left: "Idle" ("name (unnamed)") -> [w217]
    tunnel: w12 -> [w214]
    tunnel: w10 -> [w213]
    tunnel: w9 -> [w212]
    tunnel: w7 -> [w211]
    tunnel: w4 -> [w210]
    stop <- w215 stop-if-true
    n119 = case shown="\"CheckDrift\"" w217 {
      tunnel: w219 -> [_ w232 _ _ _ _]
      tunnel: ["EXIT" ("name (unnamed)") w230 "Update" ("name (unnamed)") w259 w270 w307] -> w218
      tunnel: FALSE -> [_ w229 w244 w261 w288 w344]
      tunnel: [TRUE w229 w244 w261 w288 w344] -> w215
      tunnel: w214 -> [_ _ _ _ _ w332]
      tunnel: w213 -> [_ _ _ _ _ w316]
      tunnel: w212 -> [_ _ _ _ _ w326]
      tunnel: w211 -> [_ _ _ _ _ w321]
      tunnel: w210 -> [_ _ _ _ _ w324]
      frame "EXIT" {
      }
      frame "Idle", Default {
        n120 = Dequeue Element(queue=w232, timeout in ms (-1)=-1) -> (element=w230:string)  [unwired: 1 in, 3 out]
        n121 = call "Correct Signal AE.vi"("Action"=Standard_Action_for_Focus_Lock."Read") -> ("signal out"=w227:bool)  [unwired: 1 in]
        n122 = call "Lock Control AE.vi"("Action"=Standard_Action_for_Focus_Lock."Read") -> ("Lock Control  out"=w225:T1)  [unwired: 1 in]
        n123 = Bundle By Name(cluster=w225, "Manual"=w227) -> (w224:T1)
        n124 = call "Translation Step Counter.vi"("Action"=Counter_Action."Zero") -> ()  [unwired: 1 out]
        n125 = call "Lock Control AE.vi"("Lock Control  in"=w224, "Action"=Standard_Action_for_Focus_Lock."Write") -> ()  [unwired: 1 out]
      }
      frame "Fit" {
        n126 = property on="ROI" class="IntGraph (strict)"() -> ("Value"=w242:u8[][])  [unwired: 2 in, 2 out]
        n127 = To Double Precision Float(number=w242) -> (double precision float=w241:dbl[][])
        n128 = disable-structure shown="Enabled" {
          disable-tunnel: w241 -> [w249 w254]
          disable-tunnel: [w248 w253] -> w239
          disable-tunnel: [w247 w252] -> w238
          disable-tunnel: [w246 w250] -> w235
          disable-tunnel: [w245 w251] -> w234
          frame Disabled {
            n129 = script code="addpath 'C:\\Users\\ED STED\\Documents\\Test Control Software\\Host VIs\\Focus Lock\\Matlab\\';\n[x1 y1 sx sy]=regionfit(ROI);"("ROI"=w249) -> ("x1"=w248:dbl, "y1"=w247:dbl, "sx"=w245:dbl, "sy"=w246:dbl)  [unwired: 1 in, 1 out]
          }
          frame Enabled {
            n130 = call "Locate Focal Spot.vi"("Focal Spot"=w254) -> ("sy"=w250:dbl, "sx"=w251:dbl, "cmy"=w252:dbl, "cmx"=w253:dbl)  [unwired: 7 in]
          }
        }
        n131 = Subtract(x=w234, y=w235) -> (x-y=w233:dbl)
        "Size difference History" <- w233
        n132 = Bundle("cmx"=w239, "cmy"=w238) -> (→"Position History":cluster{"cmx":dbl, "cmy":dbl})  [unwired: 1 in]
        n133 = Bundle("cmx"=w239, "cmy"=w238, w233) -> (w237:cluster{"cmx":dbl, "cmy":dbl, dbl})  [unwired: 1 in]
        n134 = call "Position AE.vi"("Current Position in"=w237, "Action"=Standard_Action_for_Position."Write Current") -> ()  [unwired: 2 in, 2 out]
      }
      frame "Update" {
        n135 = call "Lock Control AE.vi"("Action"=Standard_Action_for_Focus_Lock."Read") -> ("Lock Control  out"=w255:T1)  [unwired: 1 in]
        n136 = Unbundle By Name(w255) -> ("Lock Current"=w260:bool)
        n137 = call "Position AE.vi"("Action"=Standard_Action_for_Position."Read") -> ("Current Position out"=→"Current Position":cluster{"X":dbl, "Y":dbl, "dx - dy":dbl})  [unwired: 3 in, 1 out]
        n138 = case shown="True" w260 {
          tunnel: ["Idle" "CheckDrift"] -> w259
          frame False {
          }
          frame True {
          }
        }
      }
      frame "CheckDrift" {
        n139 = call "Position AE.vi"("Action"=Standard_Action_for_Position."Read") -> ("Locked Position out"=w285:cluster{"X":dbl, "Y":dbl, "dx - dy":dbl}, "Current Position out"=w286:cluster{"X":dbl, "Y":dbl, "dx - dy":dbl})  [unwired: 3 in]
        n140 = Cluster To Array(cluster=w286) -> (array=w283:dbl[])
        n141 = Cluster To Array(cluster=w285) -> (array=w284:dbl[])
        n142 = flat-sequence {
          tunnel: [w298] -> w282
          tunnel: w284 -> [w297]
          tunnel: w283 -> [w296]
          frame #0 {
            n143 = call-poly <vilib>:"PID.vi"("reinitialize? (F)"=TRUE, "PID gains"=T10 [{"proportional gain (Kc)"=1.0, "integral time (Ti, min)"=0.01, "derivative time (Td, min)"=0.0}, {"proportional gain (Kc)"=1.0, "integral time (Ti, min)"=0.01, "derivative time (Td, min)"=0.0}, {"proportional gain (Kc)"=1.0, "integral time (Ti, min)"=0.01, "derivative time (Td, min)"=0.0}], "process variable"=w296, "setpoint"=w297) -> ("output"=w298:dbl[])  [unwired: 6 in, 1 out]
          }
        }
        n144 = Unbundle By Name("Lock Tolorence") -> ("XY"=w280:dbl, "Z"=w279:dbl)
        n145 = Build Array(w280, w280, w279) -> (w277:dbl[])
        n146 = Absolute Value(x=w282) -> (abs(x)=w278:dbl[])
        n147 = Subtract(x=w278, y=w277) -> (x-y=w276:dbl[])
        n148 = Greater Than 0?(x=w276) -> (x > 0?=w275:bool[])
        n149 = call "Correct Signal AE.vi"("Action"=Standard_Action_for_Focus_Lock."Read") -> ("signal out"=w273:bool)  [unwired: 1 in]
        n150 = Or Array Elements(Boolean array=w275) -> (logical OR=w268:bool)
        n151 = call "Lock Control AE.vi"("Action"=Standard_Action_for_Focus_Lock."Read") -> ("Lock Control  out"=w267:T1)  [unwired: 1 in]
        n152 = Bundle By Name(cluster=w267, "Drift"=w268) -> (w265:T1)
        n153 = case shown="False" w268 {
          selector: w268 -> [w294 _]
          frame False {
            n154 = call "Lock Control AE.vi"("Action"=Standard_Action_for_Focus_Lock."Read") -> ("Lock Control  out"=w292:T1)  [unwired: 1 in]
            n155 = call "Correct Signal AE.vi"("signal in"=w294, "Action"=Standard_Action_for_Focus_Lock."Write") -> ()  [unwired: 1 out]
            n156 = Bundle By Name(cluster=w292, "Move"=FALSE) -> (w289:T1)
            n157 = call "Lock Control AE.vi"("Lock Control  in"=w289, "Action"=Standard_Action_for_Focus_Lock."Write") -> ()  [unwired: 1 out]
          }
          frame True {
          }
        }
        n158 = And(x=w268, y=w273) -> (x .and. y?=w272:bool)
        n159 = Select(t="Move", s=w272, f="Idle") -> (s? t:f=w270:string)
        n160 = call "Lock Control AE.vi"("Lock Control  in"=w265, "Action"=Standard_Action_for_Focus_Lock."Write") -> ()  [unwired: 1 out]
        "metric" <- w282
      }
      frame "Move" {
        n161 = local read "metric"() -> (w343:dbl[])
        n162 = Index Array(array=w343, index #1=0 ("index"), index #2=1 ("index"), index #3=2 ("index")) -> (element #1=w338:dbl, element #2=w333:dbl, element #3=w330:dbl)
        n163 = call "Lock Control AE.vi"("Action"=Standard_Action_for_Focus_Lock."Read") -> ("Lock Control  out"=w312:T1)  [unwired: 1 in]
        n164 = Multiply(x=-0.02, y=w333) -> (x*y=w336:dbl)
        n165 = Multiply(x=w330, y=-0.05) -> (x*y=w328:dbl)
        n166 = Multiply(x=w338, y=0.02) -> (x*y=w337:dbl)
        n167 = Build Array(w337, w336) -> (w335:dbl[])
        n168 = Build Array(w328) -> (w325:dbl[])
        n169 = Unbundle By Name(w312) -> ("EXIT"=w311:bool)
        n170 = call "AllStage_Limits_Array.vi"("Step(um)/Position(units)"=w335, "Axis"=bool[] [TRUE, TRUE], "Stage ID"=w332, "MOVE/MVR"=enum16{"MOVE", "MVR"}."MVR") -> ("Positions"=w314:dbl[], "Boolean Array"=w313:bool[], "In scale?"=w309:bool)  [unwired: 4 in, 1 out]
        n171 = call "AllStage_Limits_Array.vi"("Step(um)/Position(units)"=w325, "Axis"=w324, "Stage ID"=w326, "MOVE/MVR"=enum16{"MOVE", "MVR"}."MVR") -> ("Positions"=w319:dbl[], "Boolean Array"=w318:bool[], "In scale?"=w308:bool)  [unwired: 4 in, 1 out]
        n172 = call "P612CW.vi"("Abort"=w311, "Axis"=w313, "Positions"=w314, "Action"=StageStates."MVR", "VISA In"=w316) -> ()  [unwired: 3 in, 4 out]
        n173 = Or(x=w309, y=w308) -> (x .or. y?=w306:bool)
        n174 = call "Translation Step Counter.vi"("Action"=Counter_Action."Plus One") -> ("Num"=w304:i32)
        n175 = Less Or Equal?(x=w304, y=15) -> (x <= y?=w302:bool)
        n176 = And(x=w306, y=w302) -> (x .and. y?=w301:bool)
        n177 = call "N664CW.vi"("Velocity"=0.5, "Abort"=w311, "Axis"=w318, "Positions"=w319, "Action"=StageStates."MVR", "VISA In"=w321) -> ()  [unwired: 2 in, 4 out]
        n178 = case shown="False" w301 {
          selector: w301 -> [w352 _]
          tunnel: ["Idle" ("t") "Fit" ("t")] -> w307
          frame False {
            n179 = call "Lock Control AE.vi"("Action"=Standard_Action_for_Focus_Lock."Read") -> ("Lock Control  out"=w349:T1)  [unwired: 1 in]
            n180 = call "Correct Signal AE.vi"("signal in"=w352, "Action"=Standard_Action_for_Focus_Lock."Write") -> ()  [unwired: 1 out]
            n181 = Bundle By Name(cluster=w349, "Move"=FALSE) -> (w346:T1)
            n182 = call "Lock Control AE.vi"("Lock Control  in"=w346, "Action"=Standard_Action_for_Focus_Lock."Write") -> ()  [unwired: 1 out]
          }
          frame True {
          }
        }
        n183 = Wait Until Next ms Multiple(millisecond multiple=u32 80) -> ()  [unwired: 1 out]
      }
    }
  }
  n184 = invoke class="APTLaser" method="StopCtrl"(reference=w20, error in=w18) -> ()  [unwired: 1 in, 3 out]
